vi "delete item.vi"(10 "Index":i32, 11 "ProgramData in":T1={"Tytuły"=[], "Folder"=path "", "Data/tytul"=[], "Ostatni index"=-10, "Title"="", "Note"=""}) -> (3 "ProgramData out":T1={"Tytuły"=[], "Folder"=path "", "Data/tytul"=[], "Ostatni index"=-10, "Title"="", "Note"=""})   [LabVIEW 2020]
uses:
  #typeDef_ProgramData.ctl
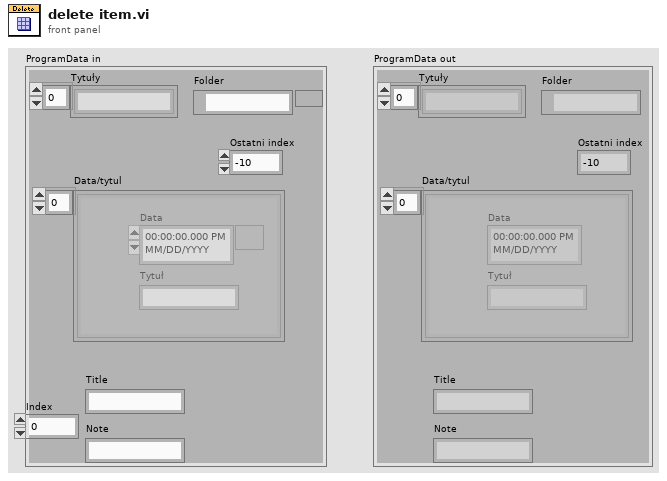
[diagram p1: front panel]
types:
  T1 = typedef "#typeDef_ProgramData.ctl" = cluster{"Tytuły":string[], "Folder":path, "Data/tytul":cluster{"Data":timestamp, "Tytuł":string}[], "Ostatni index":i32, "Title":string, "Note":string}
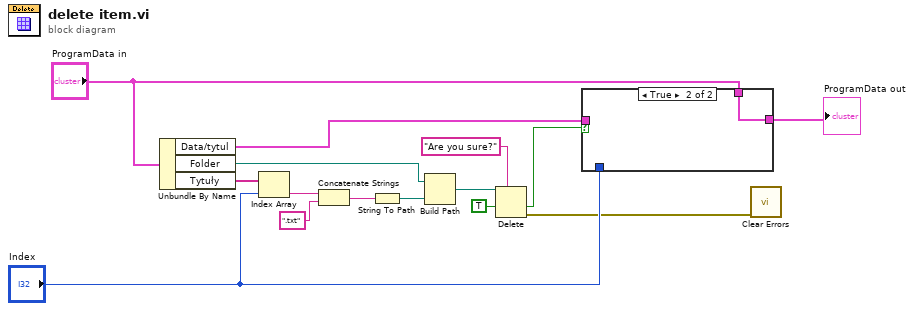
[diagram p0: block diagram]
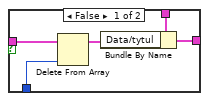
[diagram p2: hidden frame]
diagram:
  n1 = Unbundle By Name("ProgramData in") -> ("Data/tytul"=w11:cluster{"Data":timestamp, "Tytuł":string}[], "Folder"=w7:path, "Tytuły"=w2:string[])
  n2 = Index Array(array=w2, index="Index") -> (element=w3:string)
  n3 = Concatenate Strings(w3, ".txt" ("string")) -> (w5:string)
  n4 = String To Path(string=w5) -> (path=w6:path)
  n5 = Build Path(base path=w7, name or relative path=w6) -> (appended path=w12:path)
  n6 = Delete(prompt (Delete)="Are you sure?", path (use dialog)=w12, confirm (F)=TRUE) -> (cancelled=w1:bool, error out=w10:errorcluster)  [unwired: 2 in, 1 out]
  n7 = case shown="True" w1 {
    tunnel: "ProgramData in" -> [w19 w21]
    tunnel: [w18 w21] -> w14
    tunnel: "Index" -> [w17 _]
    tunnel: w11 -> [w16 _]
    frame False {
      n8 = Delete From Array(array=w16, index=w17) -> (array with subset deleted=w20:cluster{"Data":timestamp, "Tytuł":string}[])  [unwired: 1 in, 1 out]
      n9 = Bundle By Name(cluster=w19, "Data/tytul"=w20) -> (w18:T1)
    }
    frame True {
    }
  }
  "ProgramData out" <- w14
  n10 = call <vilib>:"Clear Errors.vi"("error in (no error)"=w10) -> ()  [unwired: 5 in, 2 out]
